vi "FPGA_controller.vi"() -> ()   [LabVIEW 2017]
uses:
  <vilib>/rvi/Emulation/niFpgaGetClockAttributes.vi
  <vilib>/rvi/Emulation/niFpgaSctlEmulationGetInTimedLoop.vi
  <vilib>/rvi/Emulation/niFpgaEmulationReportErrorSimple.vi
  <vilib>/rvi/eio/common/nirviEmuTemplateMethod_errors.vi
  <vilib>/rvi/Emulation/niFpgaCriticalErrorInLSC.vi
  <vilib>/eio/EIONode/EIONode.xnode
panel:
  in  "Input test":bool
  out "Translated":i16
  out "VALID":bool
  in  "Scale x2":fxp<+/-,32,16>=10.0 format="%#_21g"
  in  "m_first x2":fxp<+/-,49,33>=4.9499969482421875 format="%#_26g"
  in  "Offset x2":fxp<+/-,48,32> format="%#_26g"
  in  "1/eta x":fxp<+,8,8>=200.0 format="%#_21g"
  in  "m_first x1":fxp<+/-,49,33>=0.649993896484375 format="%#_26g"
  in  "Offset x1":fxp<+/-,48,32> format="%#_26g"
  in  "Scale x1":fxp<+/-,32,16>=5.0 format="%#_21g"
  in  "stop":bool
  # "STATES CONVERSION"
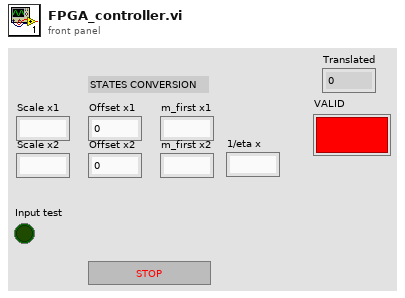
[diagram p1: front panel]
types:
  T1 = cluster{"Boolean array[0]":bool, "Boolean array[1]":bool, "Boolean array[2]":bool, "Boolean array[3]":bool, "Boolean array[4]":bool, "Boolean array[5]":bool, "Boolean array[6]":bool, "Boolean array[7]":bool, "Boolean array[8]":bool, "Boolean array[9]":bool, "Boolean array[10]":bool, "Boolean array[11]":bool, "Boolean array[12]":bool, "Boolean array[13]":bool, "Boolean array[14]":bool, "Boolean array[15]":bool}
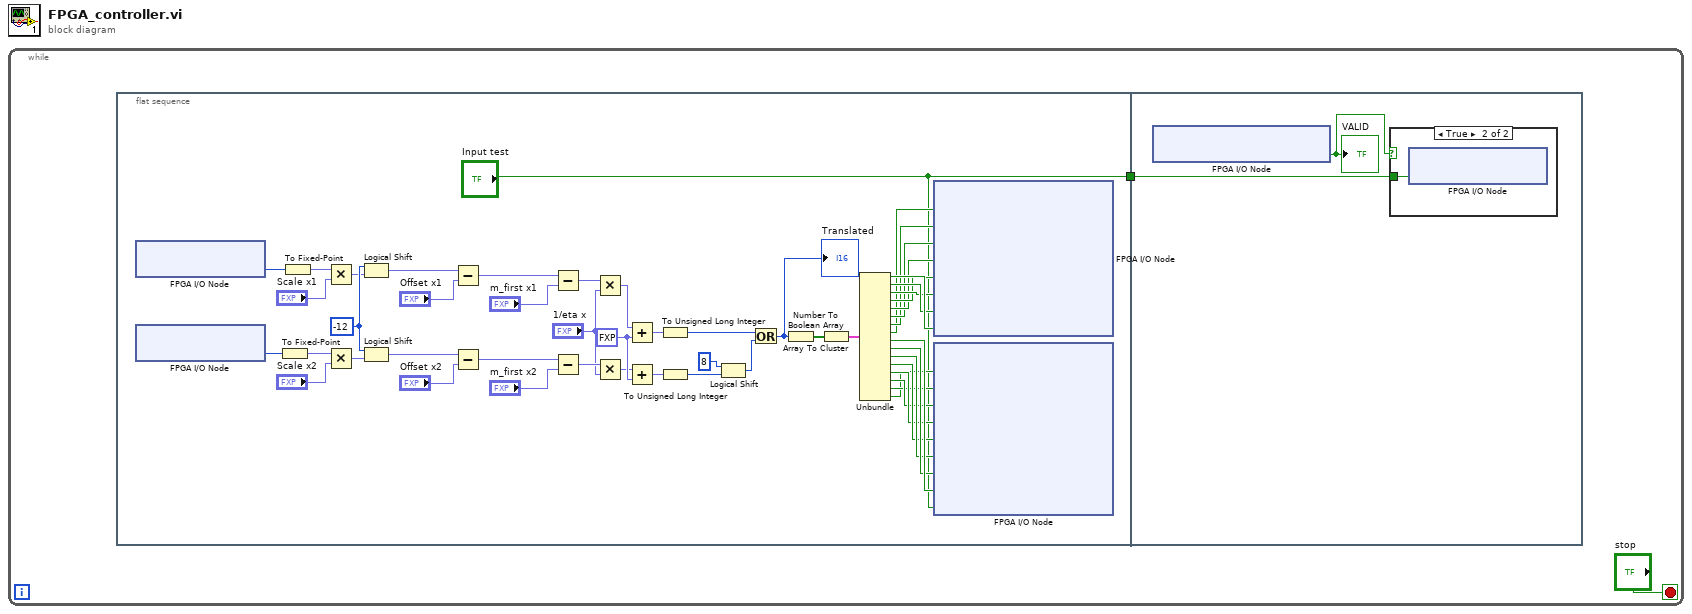
[diagram p0: block diagram]
diagram:
  n1 = while {
    stop <- "stop" stop-if-true
    n2 = flat-sequence {
      tunnel: ["Input test"] -> w1
      tunnel: w1 -> [w53]
      frame #0 {
        w29 = fxp<+,2,1> 0.5 ("y")
        w27 = i16 -12 ("y")
        n3 = xnode "FPGA I/O Node"() -> ("ConnectorA/AI0"=w6:u16)  [unwired: 1 in, 1 out]
        n4 = xnode "FPGA I/O Node"() -> ("ConnectorA/AI1"=w4:u16)  [unwired: 1 in, 1 out]
        n5 = To Fixed-Point(number=w4) -> (fixed-point=w3:fxp<+,16,16>)  [unwired: 1 in]
        n6 = To Fixed-Point(number=w6) -> (fixed-point=w5:fxp<+,16,16>)  [unwired: 1 in]
        n7 = Multiply(x=w5, y="Scale x1") -> (x*y=w26:fxp<+/-,48,32>)
        n8 = Multiply(x=w3, y="Scale x2") -> (x*y=w30:fxp<+/-,48,32>)
        n9 = Logical Shift(y=w27, x=w26) -> (x << y=w23:fxp<+/-,48,32>)
        n10 = Logical Shift(y=w27, x=w30) -> (x << y=w20:fxp<+/-,48,32>)
        n11 = Subtract(x=w23, y="Offset x1") -> (x-y=w24:fxp<+/-,49,33>)
        n12 = Subtract(x=w20, y="Offset x2") -> (x-y=w21:fxp<+/-,49,33>)
        n13 = Subtract(x=w24, y="m_first x1") -> (x-y=w25:fxp<+/-,50,34>)
        n14 = Subtract(x=w21, y="m_first x2") -> (x-y=w19:fxp<+/-,50,34>)
        n15 = Multiply(x=w25, y="1/eta x") -> (x*y=w22:fxp<+/-,58,42>)
        n16 = Multiply(x=w19, y="1/eta x") -> (x*y=w18:fxp<+/-,58,42>)
        n17 = Add(x=w22, y=w29) -> (x+y=w33:fxp<+/-,58,42>)
        n18 = Add(x=w18, y=w29) -> (x+y=w28:fxp<+/-,58,42>)
        n19 = To Unsigned Long Integer(number=w33) -> (unsigned 32bit integer=w10:u32)
        n20 = To Unsigned Long Integer(number=w28) -> (unsigned 32bit integer=w31:u32)
        n21 = Logical Shift(y=8, x=w31) -> (x << y=w9:u32)
        n22 = Or(x=w10, y=w9) -> (x .or. y?=w8:u32)
        "Translated" <- w8
        n23 = Number To Boolean Array(number=w8) -> (Boolean array=w50:bool[])
        n24 = Array To Cluster(array=w50) -> (cluster=w51:T1)
        n25 = Unbundle(w51) -> ("Boolean array[0]"=w49:bool, "Boolean array[1]"=w48:bool, "Boolean array[2]"=w47:bool, "Boolean array[3]"=w46:bool, "Boolean array[4]"=w45:bool, "Boolean array[5]"=w44:bool, "Boolean array[6]"=w43:bool, "Boolean array[7]"=w42:bool, "Boolean array[8]"=w41:bool, "Boolean array[9]"=w40:bool, "Boolean array[10]"=w39:bool, "Boolean array[11]"=w38:bool, "Boolean array[12]"=w37:bool, "Boolean array[13]"=w36:bool, "Boolean array[14]"=w35:bool, "Boolean array[15]"=w34:bool)
        n26 = xnode "FPGA I/O Node"("Component-Level IP\\pi00"=w42, "Component-Level IP\\pi01"=w43, "Component-Level IP\\pi02"=w44, "Component-Level IP\\pi03"=w45, "Component-Level IP\\pi04"=w46, "Component-Level IP\\pi05"=w47, "Component-Level IP\\pi06"=w48, "Component-Level IP\\pi07"=w49) -> ()  [unwired: 8 in, 8 out]
        n27 = xnode "FPGA I/O Node"("Component-Level IP\\pi08"=w34, "Component-Level IP\\pi09"=w35, "Component-Level IP\\pi10"=w36, "Component-Level IP\\pi11"=w37, "Component-Level IP\\pi12"=w38, "Component-Level IP\\pi13"=w39, "Component-Level IP\\pi14"=w40, "Component-Level IP\\pi15"=w41, "Component-Level IP\\pi16"="Input test") -> ()  [unwired: 9 in, 9 out]
      }
      frame #1 {
        n28 = xnode "FPGA I/O Node"() -> ("Component-Level IP\\po0"=w52:bool)  [unwired: 1 in, 1 out]
        "VALID" <- w52
        n29 = case shown="True" w52 {
          tunnel: w53 -> [_ w54]
          frame False {
          }
          frame True {
            n30 = xnode "FPGA I/O Node"("ConnectorA/DIO0"=w54) -> ()  [unwired: 1 in, 1 out]
          }
        }
      }
    }
  }
